vi "EndService (reference).vi"(1 "In":i32) -> (0 "Out":i32)   [LabVIEW 2011]
doc: "Copyright (c) 2005, Kuan Chen\nAll rights reserved.\n\nRedistribution and use in source and binary forms, with or without modification, are permitted provided that the following conditions are met:\n\n * Redistributions of source code must retain the above copyright notice, this list of conditions and the following disclaimer.\n * Redistributions in binary form must reproduce the above copyright notice, this list of conditions and the following disclaimer in the documentation and/or other materials provided with the distribution.\n * Neither the name of the Kuan Chen nor the names of its contributors may be used to endorse or promote products derived from this software without specific prior written permission.\n\nTHIS SOFTWARE IS PROVIDED BY THE COPYRIGHT HOLDERS AND CONTRIBUTORS \"AS IS\" AND ANY EXPRESS OR IMPLIED WARRANTIES, INCLUDING, BUT NOT LIMITED TO, THE IMPLIED WARRANTIES OF MERCHANTABILITY AND FITNESS FOR A PARTICULAR PURPOSE ARE DISCLAIMED. IN NO EVENT SHALL THE COPYRIGHT OWNER OR CONTRIBUTORS BE LIABLE FOR ANY DIRECT, INDIRECT, INCIDENTAL, SPECIAL, EXEMPLARY, OR CONSEQUENTIAL DAMAGES (INCLUDING, BUT NOT LIMITED TO, PROCUREMENT OF SUBSTITUTE GOODS OR SERVICES; LOSS OF USE, DATA, OR PROFITS; OR BUSINESS INTERRUPTION) HOWEVER CAUSED AND ON ANY THEORY OF LIABILITY, WHETHER IN CONTRACT, STRICT LIABILITY, OR TORT (INCLUDING NEGLIGENCE OR OTHERWISE) ARISING IN ANY WAY OUT OF THE USE OF THIS SOFTWARE, EVEN IF ADVISED OF THE POSSIBILITY OF SUCH DAMAGE.\n\nStops the OutputThread.vi from continuing to output to the output file. Returns 0."
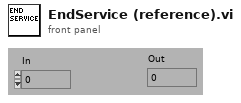
[diagram p1: front panel]
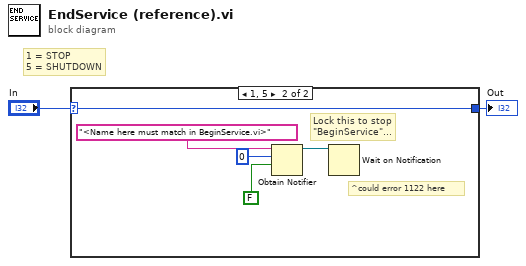
[diagram p0: block diagram]
diagram:
  # "1 = STOP\n5 = SHUTDOWN"
  n1 = case shown="1, 5" "In" {
    selector: "In" -> [w3 w4]
    tunnel: [w3 w4] -> w2
    frame 0, Default {
    }
    frame 1, 5 {
      # "^could error 1122 here"
      # "Lock this to stop\n\"BeginService\"..."
      n2 = Obtain Notifier(name (unnamed)="<Name here must match in BeginService.vi>" ("message (\"\")"), notification data type=0, create if not found? (T)=FALSE) -> (notifier out=w7:refnum<notifier>)  [unwired: 1 in, 2 out]
      n3 = Wait on Notification(notifier=w7) -> ()  [unwired: 1 in, 6 out]
    }
  }
  "Out" <- w2
